vi "Scripting - Create a New VI.vi"(8 "error in":errorcluster) -> (0 "error out":errorcluster, 3 "VI Ref Out":refnum<vi>)   [LabVIEW 2012]
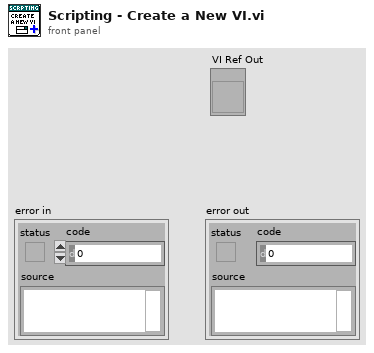
[diagram p1: front panel]
types:
  T1 = enum32{"invalid VI type", "Standard VI", "Control VI", "Global VI", "Polymorphic VI", "Configuration VI", "SubSystem", "Facade VI", "Method VI", "Statechart Diagram VI"}
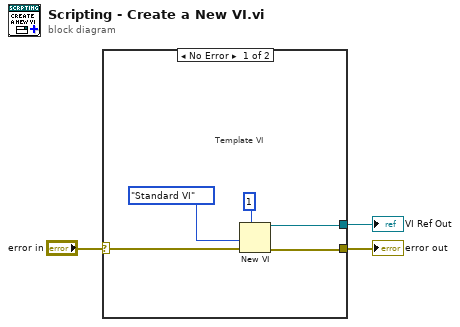
[diagram p0: block diagram]
diagram:
  n1 = case shown="No Error" "error in" {
    selector: "error in" -> [w4 w9]
    tunnel: [w8 _] -> w3
    tunnel: [w5 w9] -> w2
    frame No Error {
      # "Template VI"
      n2 = New VI(7:u32 1 ("options"), 8:w4, 9:T1."Standard VI" ("vi type (standard vi)")) -> (0:w5:errorcluster, 3:w8:refnum<vi>)  [unwired: 4 in]
    }
    frame Error {
    }
  }
  "VI Ref Out" <- w3
  "error out" <- w2
